vi "FA Forces View.vi"(11 "Model in":refnum<class "Model.lvclass">) -> ()   [LabVIEW 2016, in "M1M3SupportEUI_Views.lvlib"]
uses:
  M1M3SupportEUI_Views.lvlib
  Model/Model.lvclass
  M1M3 Support Events/M1M3 Support Events.lvclass/M1M3 Support Events.ctl
  SALLV_m1m3/DataTypes/command_ApplyOffsetForces.ctl
  SALLV_m1m3/DataTypes/command_ClearOffsetForces.ctl
  SALLV_m1m3/DataTypes/command_ApplyActiveOpticForces.ctl
  SALLV_m1m3/DataTypes/command_ClearActiveOpticForces.ctl
  SALLV_m1m3/DataTypes/command_ApplyAberrationForces.ctl
  SALLV_m1m3/DataTypes/command_ClearAberrationForces.ctl
  M1M3 Support Events/M1M3 Support Events.lvclass
  EUI Events/EUI Events.lvclass
  SALLV_m1m3/SALLV_m1m3.lvlib
panel:
  in  "ClearAberrationForcesButton":bool
  in  "ApplyAberrationForcesButton":bool
  in  "ClearActiveOpticForcesButton":bool
  in  "ApplyActiveOpticForcesButton":bool
  in  "Z441":sgl
  in  "Z440":sgl
  in  "Z443":sgl
  in  "Z442":sgl
  in  "Z401":sgl
  in  "Z431":sgl
  in  "Z430":sgl
  in  "Z439":sgl
  in  "Z438":sgl
  in  "Z437":sgl
  in  "Z436":sgl
  in  "Z435":sgl
  in  "Z434":sgl
  in  "Z433":sgl
  in  "Z432":sgl
  in  "Z421":sgl
  in  "Z420":sgl
  in  "Z429":sgl
  in  "Z428":sgl
  in  "Z427":sgl
  in  "Z426":sgl
  in  "Z425":sgl
  in  "Z424":sgl
  in  "Z423":sgl
  in  "Z422":sgl
  in  "Z411":sgl
  in  "Z410":sgl
  in  "Z419":sgl
  in  "Z418":sgl
  in  "Z417":sgl
  in  "Z416":sgl
  in  "Z415":sgl
  in  "Z414":sgl
  in  "Z413":sgl
  in  "Z412":sgl
  in  "Z409":sgl
  in  "Z408":sgl
  in  "Z407":sgl
  in  "Z406":sgl
  in  "Z405":sgl
  in  "Z404":sgl
  in  "Z403":sgl
  in  "Z402":sgl
  in  "Z341":sgl
  in  "Z340":sgl
  in  "Z343":sgl
  in  "Z342":sgl
  in  "Z301":sgl
  in  "Z331":sgl
  in  "Z330":sgl
  in  "Z339":sgl
  in  "Z338":sgl
  in  "Z337":sgl
  in  "Z336":sgl
  in  "Z335":sgl
  in  "Z334":sgl
  in  "Z333":sgl
  in  "Z332":sgl
  in  "Z321":sgl
  in  "Z320":sgl
  in  "Z329":sgl
  in  "Z328":sgl
  in  "Z327":sgl
  in  "Z326":sgl
  in  "Z325":sgl
  in  "Z324":sgl
  in  "Z323":sgl
  in  "Z322":sgl
  in  "Z311":sgl
  in  "Z310":sgl
  in  "Z319":sgl
  in  "Z318":sgl
  in  "Z317":sgl
  in  "Z316":sgl
  in  "Z315":sgl
  in  "Z314":sgl
  in  "Z313":sgl
  in  "Z312":sgl
  in  "Z309":sgl
  in  "Z308":sgl
  in  "Z307":sgl
  in  "Z306":sgl
  in  "Z305":sgl
  in  "Z304":sgl
  in  "Z303":sgl
  in  "Z302":sgl
  in  "Z241":sgl
  in  "Z240":sgl
  in  "Z243":sgl
  in  "Z242":sgl
  in  "Z201":sgl
  in  "Z231":sgl
  in  "Z230":sgl
  in  "Z239":sgl
  in  "Z238":sgl
  in  "Z237":sgl
  in  "Z236":sgl
  in  "Z235":sgl
  in  "Z234":sgl
  in  "Z233":sgl
  in  "Z232":sgl
  in  "Z221":sgl
  in  "Z220":sgl
  in  "Z229":sgl
  in  "Z228":sgl
  in  "Z227":sgl
  in  "Z226":sgl
  in  "Z225":sgl
  in  "Z224":sgl
  in  "Z223":sgl
  in  "Z222":sgl
  in  "Z211":sgl
  in  "Z210":sgl
  in  "Z219":sgl
  in  "Z218":sgl
  in  "Z217":sgl
  in  "Z216":sgl
  in  "Z215":sgl
  in  "Z214":sgl
  in  "Z213":sgl
  in  "Z212":sgl
  in  "Z209":sgl
  in  "Z208":sgl
  in  "Z207":sgl
  in  "Z206":sgl
  in  "Z205":sgl
  in  "Z204":sgl
  in  "Z203":sgl
  in  "Z202":sgl
  in  "Y430":sgl
  in  "Y438":sgl
  in  "Y437":sgl
  in  "Y434":sgl
  in  "Y433":sgl
  in  "Y432":sgl
  in  "Y421":sgl
  in  "Y420":sgl
  in  "Y429":sgl
  in  "Y427":sgl
  in  "Y424":sgl
  in  "Y423":sgl
  in  "Y422":sgl
  in  "Y411":sgl
  in  "Y410":sgl
  in  "Y418":sgl
  in  "Y417":sgl
  in  "Y416":sgl
  in  "Y415":sgl
  in  "Y414":sgl
  in  "Y409":sgl
  in  "Y408":sgl
  in  "Y230":sgl
  in  "Y238":sgl
  in  "Y237":sgl
  in  "Y234":sgl
  in  "Y233":sgl
  in  "Y232":sgl
  in  "Y221":sgl
  in  "Y220":sgl
  in  "Y229":sgl
  in  "Y227":sgl
  in  "Y224":sgl
  in  "Y223":sgl
  in  "Y222":sgl
  in  "Y211":sgl
  in  "Y210":sgl
  in  "Y218":sgl
  in  "Y217":sgl
  in  "Y216":sgl
  in  "Y215":sgl
  in  "Y214":sgl
  in  "Y209":sgl
  in  "Y208":sgl
  in  "Y330":sgl
  in  "Y338":sgl
  in  "Y337":sgl
  in  "Y334":sgl
  in  "Y333":sgl
  in  "Y332":sgl
  in  "Y321":sgl
  in  "Y320":sgl
  in  "Y329":sgl
  in  "Y327":sgl
  in  "Y326":sgl
  in  "Y324":sgl
  in  "Y323":sgl
  in  "Y322":sgl
  in  "Y311":sgl
  in  "Y310":sgl
  in  "Y318":sgl
  in  "Y317":sgl
  in  "Y316":sgl
  in  "Y315":sgl
  in  "Y314":sgl
  in  "Y313":sgl
  in  "Y309":sgl
  in  "Y308":sgl
  in  "Y305":sgl
  in  "Y304":sgl
  in  "Y303":sgl
  in  "Y302":sgl
  in  "Z141":sgl
  in  "Z140":sgl
  in  "Z143":sgl
  in  "Z142":sgl
  in  "Z101":sgl
  in  "Z131":sgl
  in  "Z130":sgl
  in  "Z139":sgl
  in  "Z138":sgl
  in  "Z137":sgl
  in  "Z136":sgl
  in  "Z135":sgl
  in  "Z134":sgl
  in  "Z133":sgl
  in  "Z132":sgl
  in  "Z121":sgl
  in  "Z120":sgl
  in  "Z129":sgl
  in  "Z128":sgl
  in  "Z127":sgl
  in  "Z126":sgl
  in  "Z125":sgl
  in  "Z124":sgl
  in  "Z123":sgl
  in  "Z122":sgl
  in  "Z111":sgl
  in  "Z110":sgl
  in  "Z119":sgl
  in  "Z118":sgl
  in  "Z117":sgl
  in  "Z116":sgl
  in  "Z115":sgl
  in  "Z114":sgl
  in  "Z113":sgl
  in  "Z112":sgl
  in  "Z109":sgl
  in  "Z108":sgl
  in  "Z107":sgl
  in  "Z106":sgl
  in  "Z105":sgl
  in  "Z104":sgl
  in  "Z103":sgl
  in  "Z102":sgl
  in  "Y130":sgl
  in  "Y138":sgl
  in  "Y137":sgl
  in  "Y134":sgl
  in  "Y133":sgl
  in  "Y132":sgl
  in  "Y121":sgl
  in  "Y120":sgl
  in  "Y129":sgl
  in  "Y127":sgl
  in  "Y126":sgl
  in  "Y124":sgl
  in  "Y123":sgl
  in  "Y122":sgl
  in  "Y111":sgl
  in  "Y110":sgl
  in  "Y118":sgl
  in  "Y117":sgl
  in  "Y116":sgl
  in  "Y115":sgl
  in  "Y114":sgl
  in  "Y113":sgl
  in  "Y109":sgl
  in  "Y108":sgl
  in  "Y105":sgl
  in  "Y104":sgl
  in  "Y103":sgl
  in  "ClearForcesButton":bool
  in  "ApplyOffsetForcesButton":bool
  in  "Y102":sgl
  in  "X435":sgl
  in  "X428":sgl
  in  "X412":sgl
  in  "X335":sgl
  in  "X328":sgl
  in  "X312":sgl
  in  "X235":sgl
  in  "X228":sgl
  in  "X212":sgl
  in  "X135":sgl
  in  "X128":sgl
  in  "X112":sgl
  # "Force Actuator\nApply Forces"
  # "Z"
  # "Y"
  # "0"
  # "1"
  # "2"
  # "3"
  # "4"
  # "5"
  # "6"
  # "7"
  # "8"
  # "9"
  # "0"
  # "1"
  # "2"
  # "3"
  # "4"
  # "5"
  # "6"
  # "7"
  # "8"
  # "9"
  # "100"
  # "100"
  # "110"
  # "110"
  # "X"
  # "120"
  # "120"
  # "112"
  # "212"
  # "130"
  # "130"
  # "128"
  # "228"
  # "140"
  # "140"
  # "135"
  # "235"
  # "200"
  # "200"
  # "210"
  # "312"
  # "210"
  # "412"
  # "220"
  # "220"
  # "328"
  # "428"
  # "230"
  # "230"
  # "335"
  # "435"
  # "240"
  # "240"
  # "300"
  # "300"
  # "310"
  # "310"
  # "320"
  # "320"
  # "330"
  # "330"
  # "340"
  # "340"
  # "400"
  # "400"
  # "410"
  # "410"
  # "420"
  # "420"
  # "430"
  # "430"
  # "440"
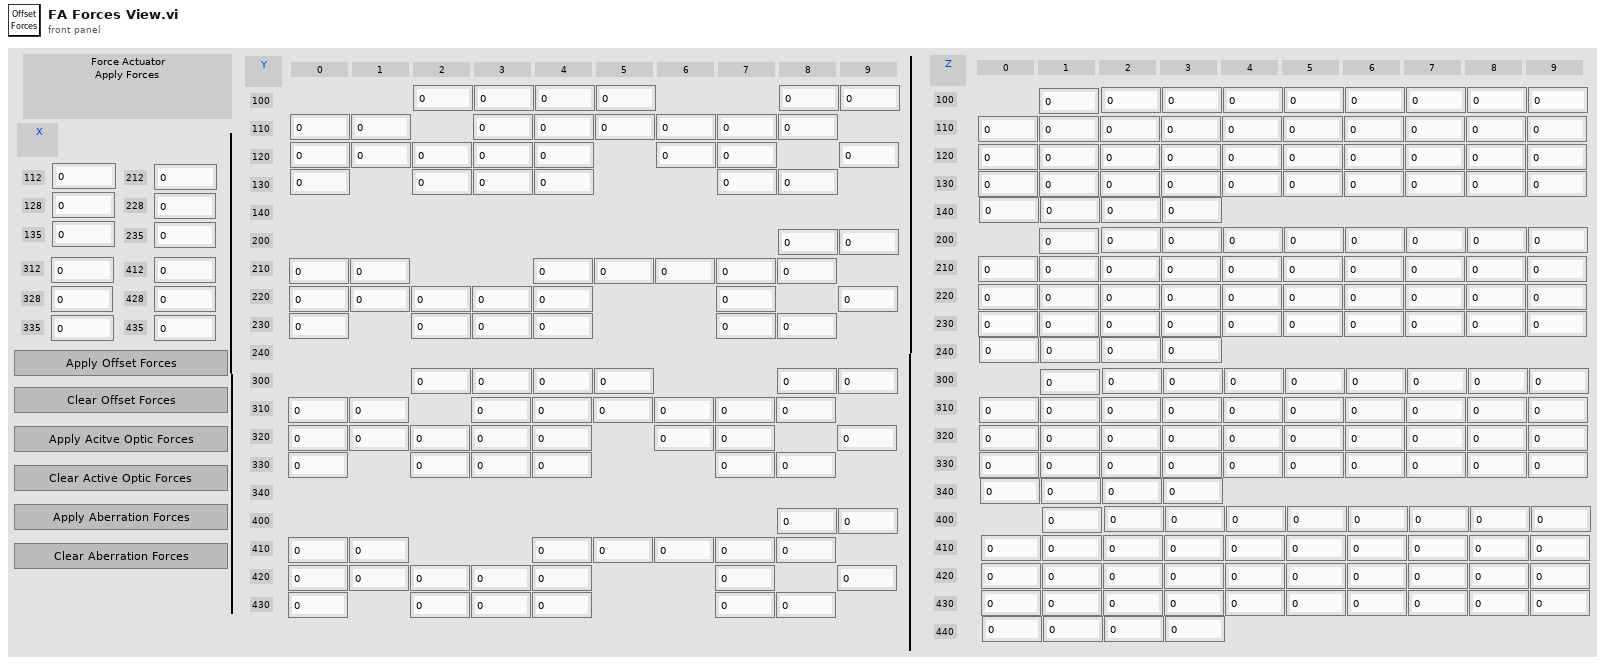
[diagram p1: front panel]
types:
  T1 = typedef "M1M3SupportEUI_TypeDefs.lvlib/M1M3 Support Events.ctl" = cluster{"Inclinometer  Data":refnum<user-event>, "IMS Data":refnum<user-event>, "SAL Connected":refnum<user-event>, "Accelerometer Data":refnum<user-event>, "OuterLoop Data":refnum<user-event>, "ErrorCode Event":refnum<user-event>, "InterlockStatus Event":refnum<user-event>, "InterlockWarning Event":refnum<user-event>, "Gyro Data":refnum<user-event>, "HP Actuator Info Event":refnum<user-event>, " FA Info Event":refnum<user-event>, "HP Monitor Info Event":refnum<user-event>, "FA Data":refnum<user-event>, "HP Actuator data":refnum<user-event>, "HP Monitor data":refnum<user-event>, "Air Supply Status Event":refnum<user-event>, "Air Supply Warning Event":refnum<user-event>, "Power Data":refnum<user-event>, "PID Data":refnum<user-event>, "PID Info Event":refnum<user-event>, "Power Status Event":refnum<user-event>, "Power Supply Status Event":refnum<user-event>, "Power Warning Event":refnum<user-event>, "Summary State Event":refnum<user-event>, "Detailed State Event":refnum<user-event>, "FA Force Warning Event":refnum<user-event>, "FA Warning Event":refnum<user-event>, "FA State Event":refnum<user-event>, "Applied AberrationForces Event":refnum<user-event>, "Applied Acceleration Forcces Event":refnum<user-event>, "Applied Azimuth Forces Event":refnum<user-event>, "Applied Active Optic Forces Event":refnum<user-event>, "Applied Balance Forces Event":refnum<user-event>, "Applied Cylinder Forces Event":refnum<user-event>, "Applied Elevation Forces Event":refnum<user-event>, "Applied Forces Event":refnum<user-event>, "Applied Offset Forces Event":refnum<user-event>, "Applied Static Forces Event":refnum<user-event>, "Applied Thermal Forces Event":refnum<user-event>, "Applied Velocity Forces Event":refnum<user-event>, "Rejected Aberration Force Event":refnum<user-event>, "Rejected Acceleration Forces Event":refnum<user-event>, "Rejected Active Optic Forces Event":refnum<user-event>, "Rejected Azimuth Forces Event":refnum<user-event>, "Rejected Balance Forces Event":refnum<user-event>, "Rejected Cylinder Forces Event":refnum<user-event>, "Rejected Elevation Forces Event":refnum<user-event>, "Rejected Forces Event":refnum<user-event>, "Rejected Offset Forces Event":refnum<user-event>, "Rejected Static Forces Event":refnum<user-event>, "Rejected Thermal Forces Event":refnum<user-event>, "Rejected Velocity Forces Event":refnum<user-event>, "Command Rejection Event":refnum<user-event>, "Setting Verions Event":refnum<user-event>, "Settings Applied Event":refnum<user-event>}
  T2 = enum16{"", "DetailedState_DetailedStates_DisabledState", "DetailedState_DetailedStates_EnabledState", "DetailedState_DetailedStates_FaultState", "DetailedState_DetailedStates_OfflineState", "DetailedState_DetailedStates_StandbyState", "DetailedState_DetailedStates_ParkedState", "DetailedState_DetailedStates_RaisingState", "DetailedState_DetailedStates_ActiveState", "DetailedState_DetailedStates_LoweringState", "DetailedState_DetailedStates_EngineeringState", "DetailedState_DetailedStates_ParkedEngineeringState", "DetailedState_DetailedStates_RaisingEngineeringState", "DetailedState_DetailedStates_ActiveEngineeringState", "DetailedState_DetailedStates_LoweringEngineeringState", "DetailedState_DetailedStates_LoweringFaultState", "DetailedState_DetailedStates_ProfileHardpointCorrectionState"}
  T3 = typedef "SALLV_m1m3.lvlib/command_ApplyOffsetForces.ctl" = cluster{"XForces[12]":sgl[], "YForces[100]":sgl[], "ZForces[156]":sgl[]}
  T4 = typedef "SALLV_m1m3.lvlib/command_ClearOffsetForces.ctl" = cluster{"ClearOffsetForces":bool}
  T5 = typedef "SALLV_m1m3.lvlib/command_ApplyActiveOpticForces.ctl" = cluster{"ZForces[156]":sgl[]}
  T6 = typedef "SALLV_m1m3.lvlib/command_ClearActiveOpticForces.ctl" = cluster{"ClearActiveOpticForces":bool}
  T7 = typedef "SALLV_m1m3.lvlib/command_ApplyAberrationForces.ctl" = cluster{"ZForces[156]":sgl[]}
  T8 = typedef "SALLV_m1m3.lvlib/command_ClearAberrationForces.ctl" = cluster{"ClearAberrationForces":bool}
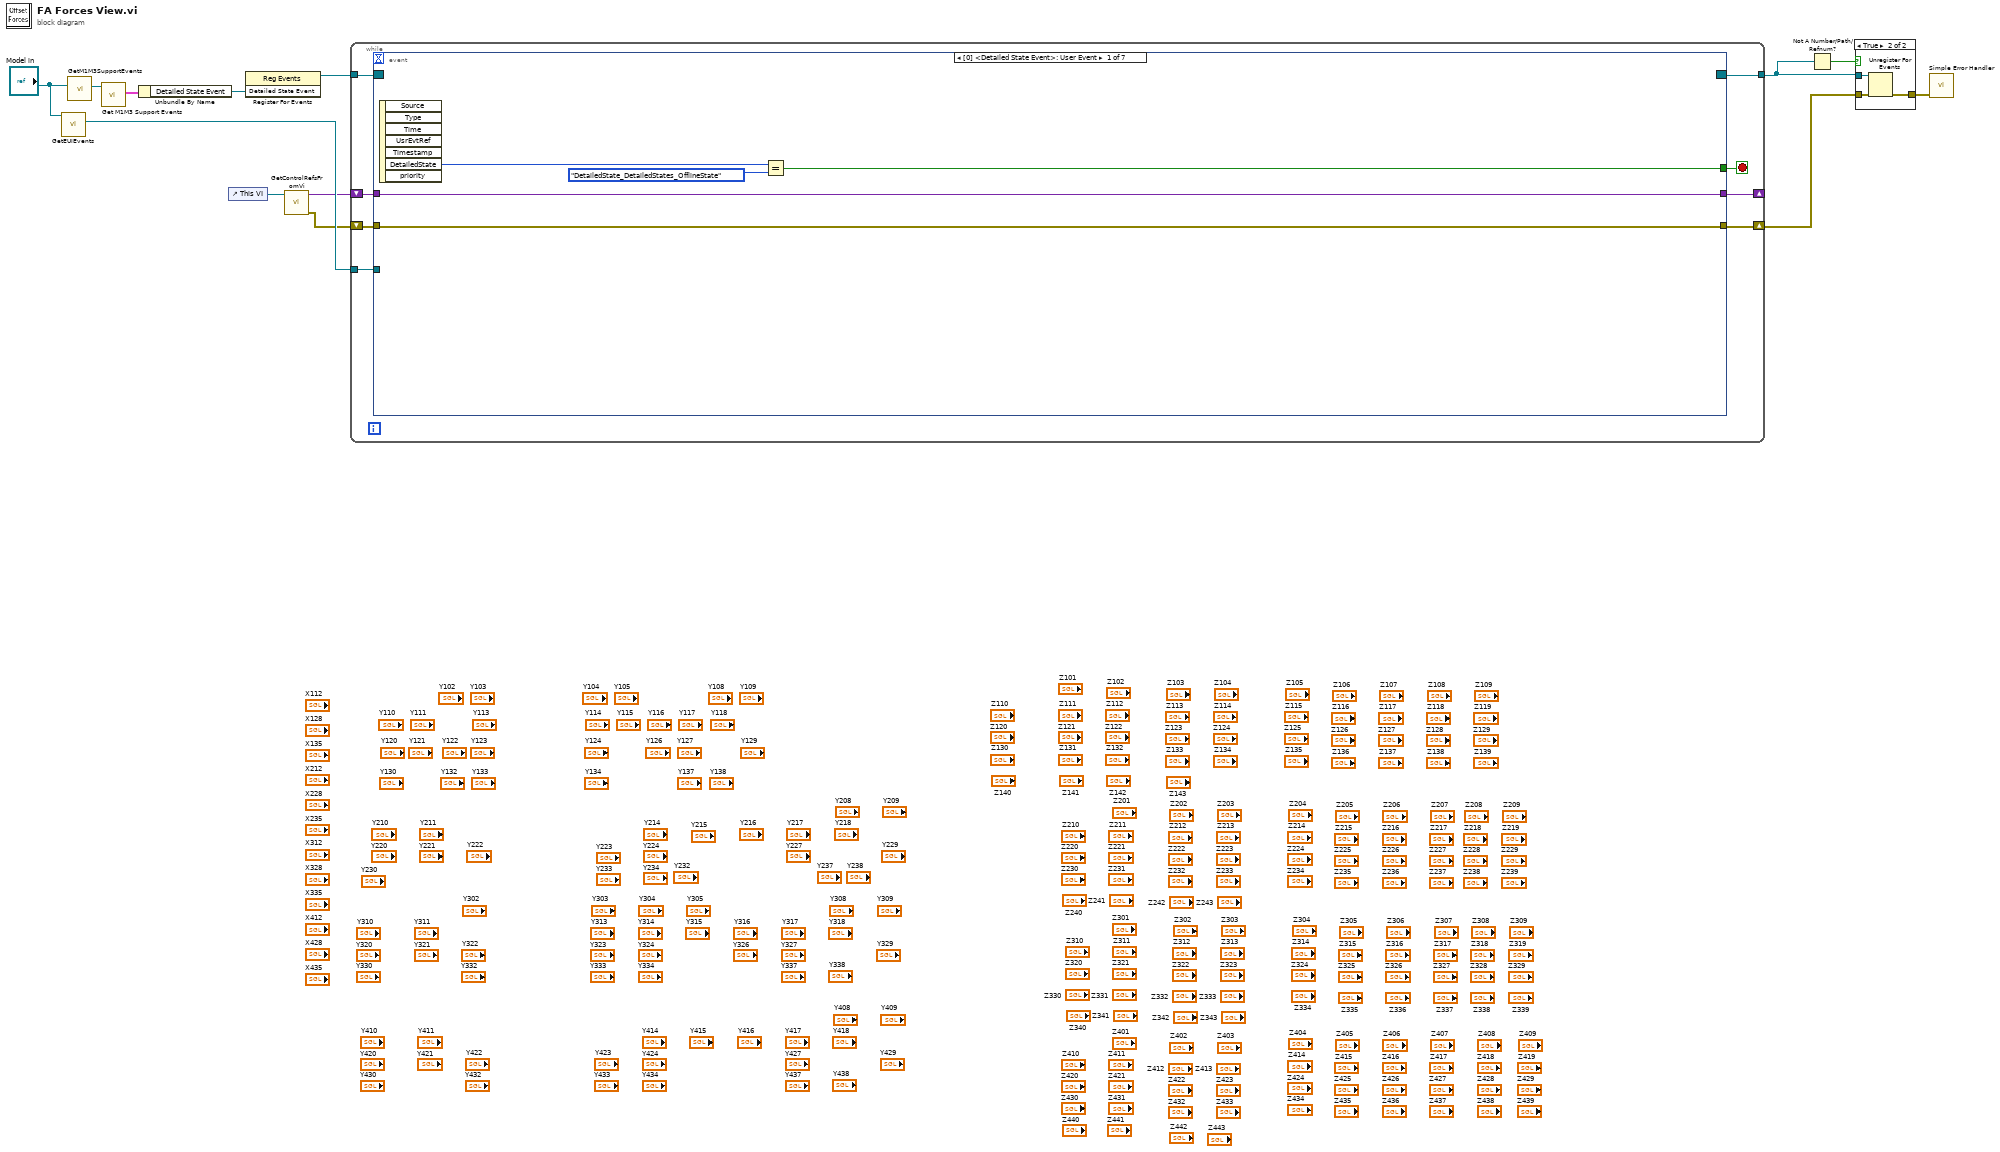
[diagram p0: block diagram]
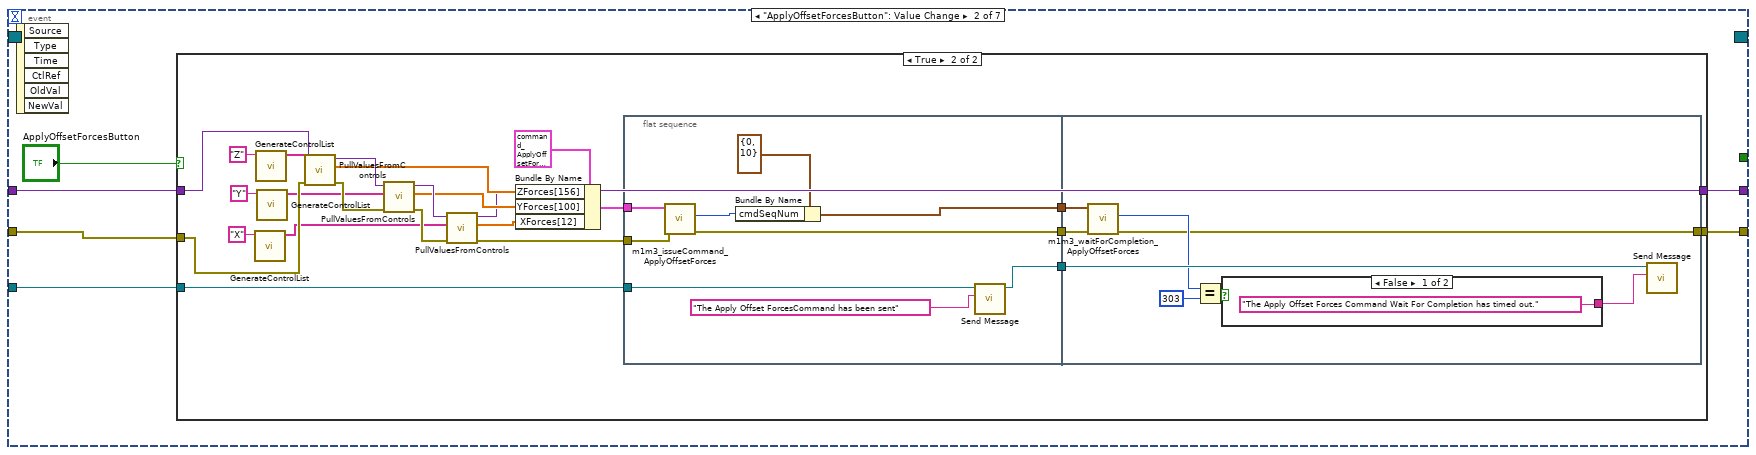
[diagram p2: hidden frame]
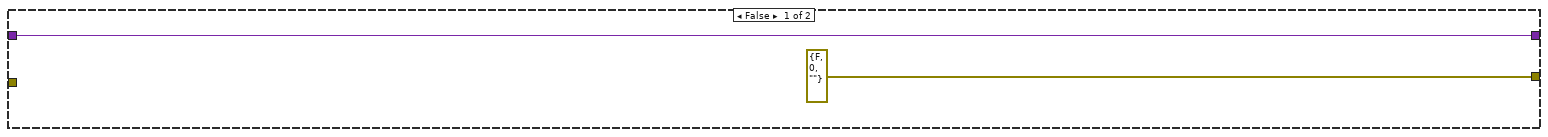
[diagram p3: hidden frame]
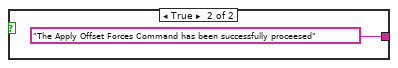
[diagram p4: hidden frame]
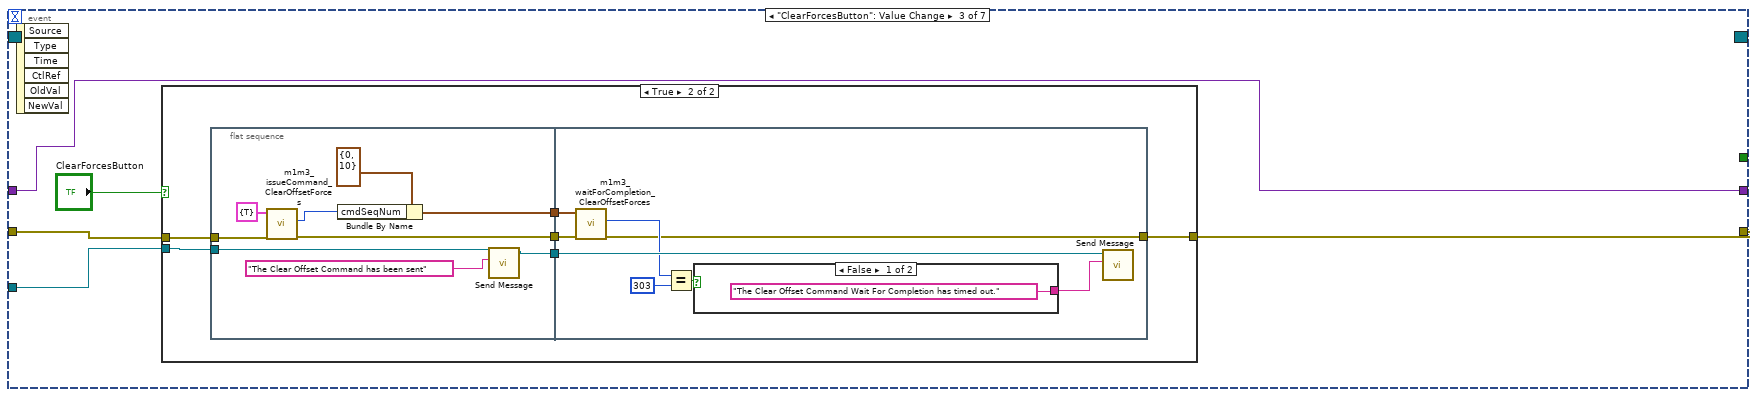
[diagram p5: hidden frame]
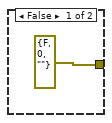
[diagram p6: hidden frame]
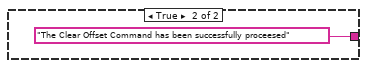
[diagram p7: hidden frame]
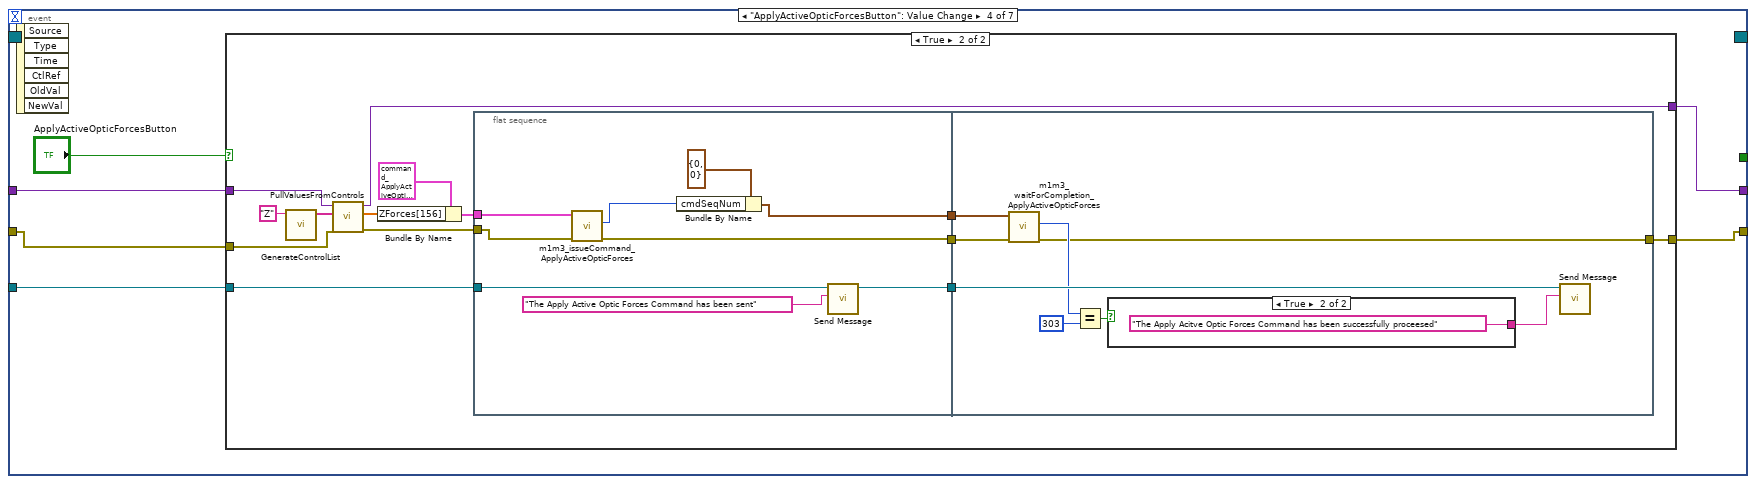
[diagram p8: hidden frame]
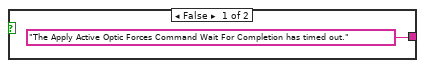
[diagram p10: hidden frame]
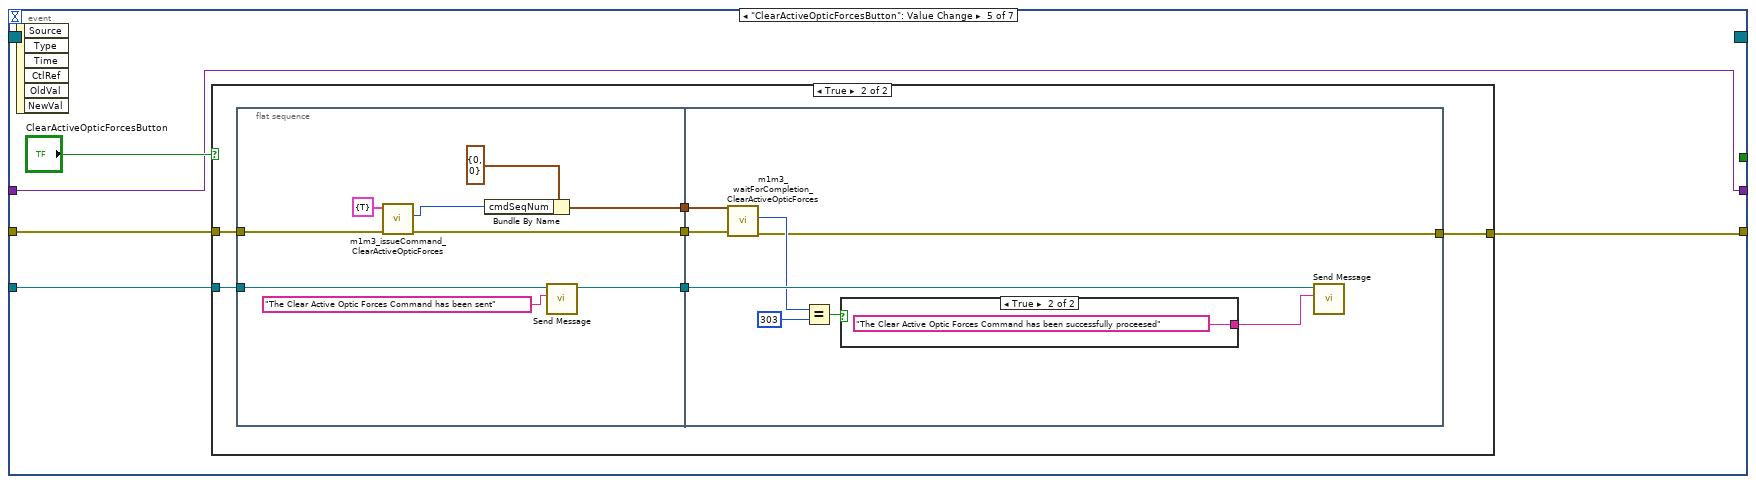
[diagram p11: hidden frame]
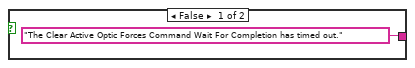
[diagram p13: hidden frame]
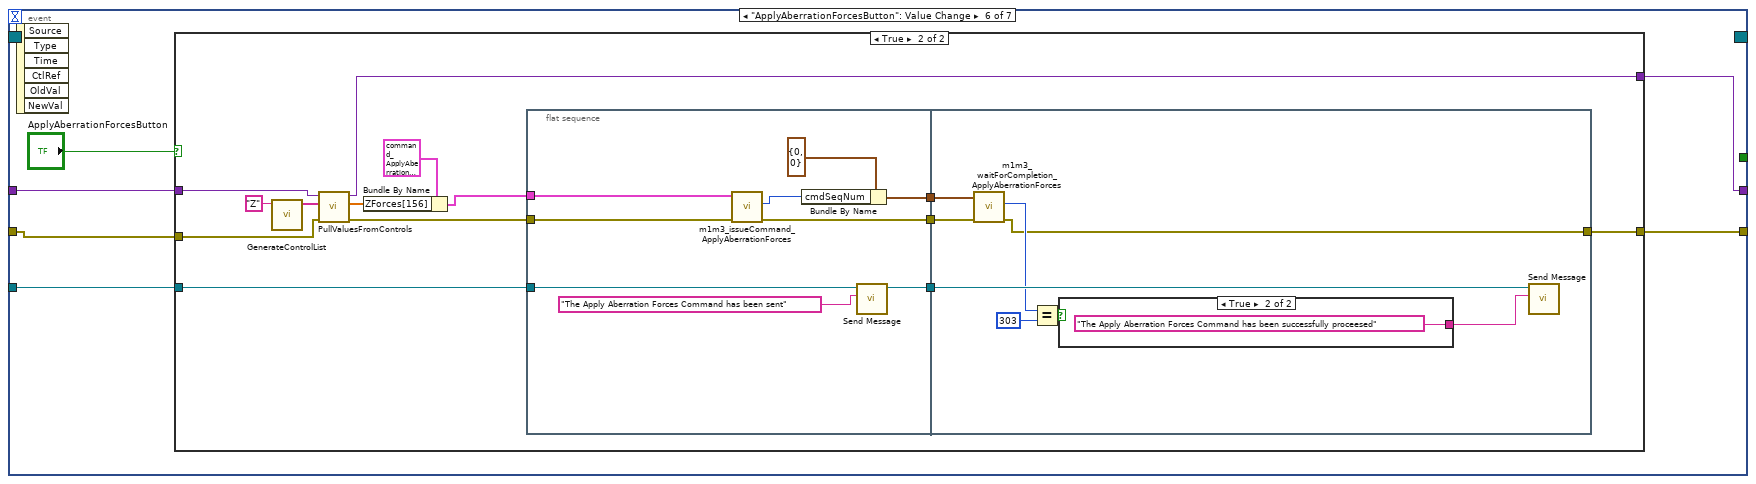
[diagram p14: hidden frame]
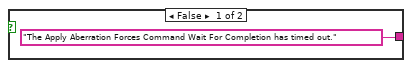
[diagram p16: hidden frame]
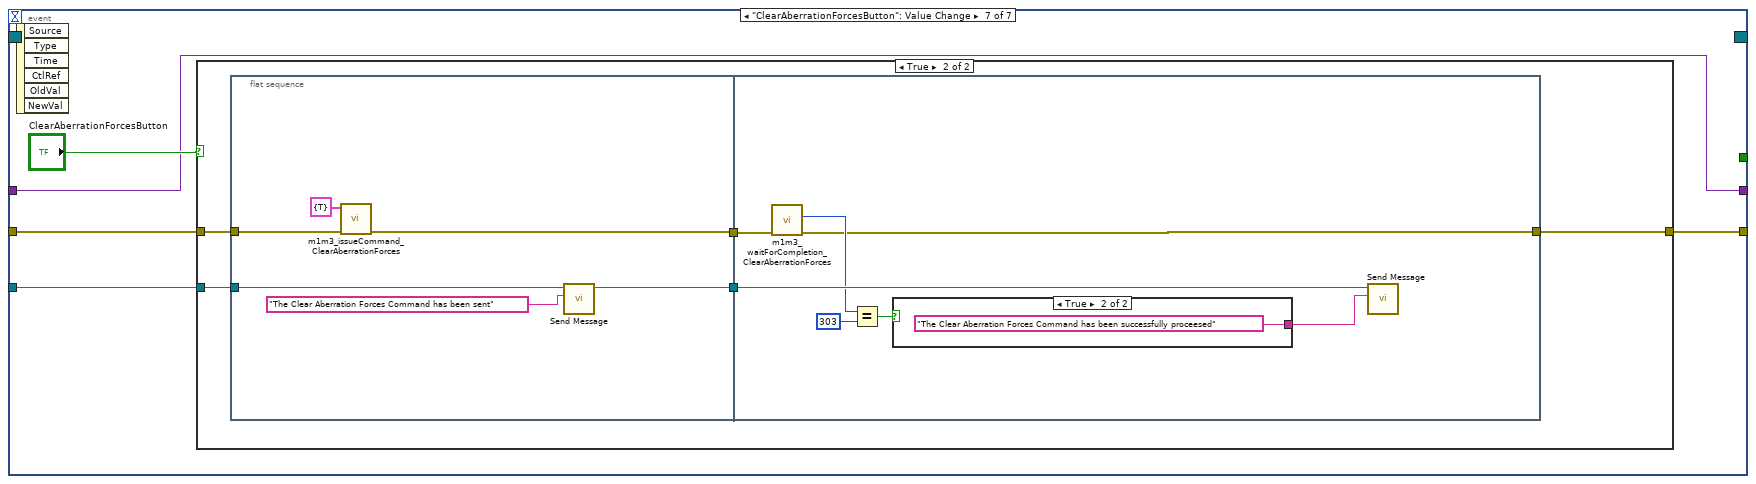
[diagram p17: hidden frame]
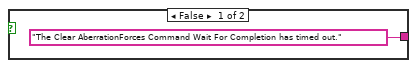
[diagram p19: hidden frame]
diagram:
  n1 = call "GetEUIEvents.vi"("Model in"="Model in") -> ("EUI Events out"=w5:refnum<class "EUI Events.lvclass">)  [unwired: 8 in, 2 out]
  n2 = call "GetM1M3SupportEvents.vi"("Model in"="Model in") -> ("M1M3 Support Events out"=w12:refnum<class "M1M3 Support Events.lvclass">)  [unwired: 8 in, 2 out]
  n3 = call "Get M1M3 Support Events.vi"("M1M3 Support Events in"=w12) -> ("M1M3 Support Events"=w11:T1)  [unwired: 9 in, 1 out]
  n4 = Unbundle By Name(w11) -> ("Detailed State Event"=w13:refnum<user-event>)
  n5 = control-ref of="This VI"() -> (w3:refnum<vi>)
  n6 = register-events(w13) -> (reference out=w10:refnum<event-registration>)  [unwired: 2 in, 1 out]
  n7 = call "GetControlRefsFromVi.vi"("VI Refnum"=w3) -> ("error out"=w1:errorcluster, "Variant"=w2:variant)  [unwired: 9 in]
  n8 = while {
    tunnel: w10 -> [w21]
    tunnel: [w20] -> w7
    tunnel: w5 -> [w18]
    shift-right: [w15] -> _
    shift-left: w2 -> [w17]
    shift-right: [w14] -> w4
    shift-left: w1 -> [w16]
    stop <- w19 stop-if-true
    n9 = event shown="[0] <Detailed State Event>: User Event" {
      selector: w21 -> [_ _ _ _ _ _ _]
      dyn-events: [_ _ _ _ _ _ _] -> w20
      timeout: _ -> [_ _ _ _ _ _ _]
      tunnel: [w24 _ _ _ _ _ _] -> w19
      tunnel: w18 -> [_ w31 w81 w111 w152 w185 w225]
      tunnel: [w22 w30 w80 w109 w150 w182 w222] -> w14
      tunnel: w17 -> [w23 w29 w79 w113 w153 w184 w224]
      tunnel: w16 -> [w22 w28 w78 w112 w151 w183 w223]
      tunnel: [w23 w27 w79 w110 w153 w181 w224] -> w15
      event User Event {
        n10 = event-data() -> ("DetailedState"=w25:T2)  [unwired: 1 in, 6 out]
        n11 = Equal?(x=w25, y=T2."DetailedState_DetailedStates_OfflineState") -> (x = y?=w24:bool)
      }
      event "ApplyOffsetForcesButton": Value Change {
        n12 = event-data() -> ()  [unwired: 1 in, 6 out]
        n13 = case shown="True" "ApplyOffsetForcesButton" {
          tunnel: w31 -> [_ w58]
          tunnel: [errorcluster {"status"=FALSE, "code"=0, "source"=""} ("error constant") w52] -> w30
          tunnel: w29 -> [w33 w51]
          tunnel: w28 -> [_ w50]
          tunnel: [w33 w41] -> w27
          frame False {
          }
          frame True {
            n14 = call "GenerateControlList.vi"("ListType"="X") -> ("ControlList"=w35:string[])  [unwired: 10 in]
            n15 = call "GenerateControlList.vi"("ListType"="Z") -> ("ControlList"=w37:string[])  [unwired: 10 in]
            n16 = call "GenerateControlList.vi"("ListType"="Y") -> ("ControlList"=w36:string[])  [unwired: 10 in]
            n17 = call "PullValuesFromControls.vi"("error in (no error)"=w50, "ControlNameArray"=w37, "Variant In"=w51) -> ("error out"=w48:errorcluster, "ControlValuesArray"=w43:sgl[], "Variant out"=w49:variant)  [unwired: 6 in]
            n18 = call "PullValuesFromControls.vi"("error in (no error)"=w48, "ControlNameArray"=w36, "Variant In"=w49) -> ("error out"=w47:errorcluster, "ControlValuesArray"=w44:sgl[], "Variant out"=w46:variant)  [unwired: 6 in]
            n19 = call "PullValuesFromControls.vi"("error in (no error)"=w47, "ControlNameArray"=w35, "Variant In"=w46) -> ("error out"=w42:errorcluster, "ControlValuesArray"=w45:sgl[], "Variant out"=w41:variant)  [unwired: 6 in]
            n20 = Bundle By Name(cluster=T3 {"XForces[12]"=[0.0, 0.0, 0.0, 0.0, 0.0, 0.0, 0.0, 0.0, 0.0, 0.0, 0.0, 0.0], "YForces[100]"=[0.0, 0.0, 0.0, 0.0, 0.0, 0.0, 0.0, 0.0, 0.0, 0.0, 0.0, 0.0, 0.0, 0.0, 0.0, 0.0, 0.0, 0.0, 0.0, 0.0, 0.0, 0.0, 0.0, 0.0, 0.0, 0.0, 0.0, 0.0, 0.0, 0.0, 0.0, 0.0, 0.0, 0.0, 0.0, 0.0, 0.0, 0.0, 0.0, 0.0, 0.0, 0.0, 0.0, 0.0, 0.0, 0.0, 0.0, 0.0, 0.0, 0.0, 0.0, 0.0, 0.0, 0.0, 0.0, 0.0, 0.0, 0.0, 0.0, 0.0, 0.0, 0.0, 0.0, 0.0, 0.0, 0.0, 0.0, 0.0, 0.0, 0.0, 0.0, 0.0, 0.0, 0.0, 0.0, 0.0, 0.0, 0.0, 0.0, 0.0, 0.0, 0.0, 0.0, 0.0, 0.0, 0.0, 0.0, 0.0, 0.0, 0.0, 0.0, 0.0, 0.0, 0.0, 0.0, 0.0, 0.0, 0.0, 0.0, 0.0], "ZForces[156]"=[0.0, 0.0, 0.0, 0.0, 0.0, 0.0, 0.0, 0.0, 0.0, 0.0, 0.0, 0.0, 0.0, 0.0, 0.0, 0.0, 0.0, 0.0, 0.0, 0.0, 0.0, 0.0, 0.0, 0.0, 0.0, 0.0, 0.0, 0.0, 0.0, 0.0, 0.0, 0.0, 0.0, 0.0, 0.0, 0.0, 0.0, 0.0, 0.0, 0.0, 0.0, 0.0, 0.0, 0.0, 0.0, 0.0, 0.0, 0.0, 0.0, 0.0, 0.0, 0.0, 0.0, 0.0, 0.0, 0.0, 0.0, 0.0, 0.0, 0.0, 0.0, 0.0, 0.0, 0.0, 0.0, 0.0, 0.0, 0.0, 0.0, 0.0, 0.0, 0.0, 0.0, 0.0, 0.0, 0.0, 0.0, 0.0, 0.0, 0.0, 0.0, 0.0, 0.0, 0.0, 0.0, 0.0, 0.0, 0.0, 0.0, 0.0, 0.0, 0.0, 0.0, 0.0, 0.0, 0.0, 0.0, 0.0, 0.0, 0.0, 0.0, 0.0, 0.0, 0.0, 0.0, 0.0, 0.0, 0.0, 0.0, 0.0, 0.0, 0.0, 0.0, 0.0, 0.0, 0.0, 0.0, 0.0, 0.0, 0.0, 0.0, 0.0, 0.0, 0.0, 0.0, 0.0, 0.0, 0.0, 0.0, 0.0, 0.0, 0.0, 0.0, 0.0, 0.0, 0.0, 0.0, 0.0, 0.0, 0.0, 0.0, 0.0, 0.0, 0.0, 0.0, 0.0, 0.0, 0.0, 0.0, 0.0, 0.0, 0.0, 0.0, 0.0, 0.0, 0.0]} ("command_ApplyOffsetForces_Ctl"), "ZForces[156]"=w43, "YForces[100]"=w44, "XForces[12]"=w45) -> (w55:T3)
            n21 = flat-sequence {
              tunnel: w58 -> [w67]
              tunnel: [w65] -> w57
              tunnel: w55 -> [w64]
              tunnel: w42 -> [w63]
              tunnel: [w60] -> w54
              tunnel: [w59] -> w53
              tunnel: w57 -> [w72]
              tunnel: w54 -> [w71]
              tunnel: w53 -> [w70]
              tunnel: [w68] -> w52
              frame #0 {
                n22 = call "m1m3_issueCommand_ApplyOffsetForces.vi"("error in (no error)"=w63, "command_ApplyOffsetForces_Ctl"=w64) -> ("error out"=w60:errorcluster, "function return"=w61:i32)  [unwired: 7 in, 1 out]
                n23 = Bundle By Name(cluster=cluster{"cmdSeqNum":i32, "timeout":u32} {"cmdSeqNum"=0, "timeout"=10} ("waitComplete_Ctl"), "cmdSeqNum"=w61) -> (w59:cluster{"cmdSeqNum":i32, "timeout":u32})
                n24 = call "Send Message.vi"("Message"="The Apply Offset ForcesCommand has been sent", "EUI Events in"=w67) -> ("EUI Events out"=w65:refnum<class "EUI Events.lvclass">)  [unwired: 8 in, 1 out]
              }
              frame #1 {
                n25 = call "m1m3_waitForCompletion_ApplyOffsetForces.vi"("error in (no error)"=w71, "waitComplete_Ctl"=w70) -> ("error out"=w68:errorcluster, "function return"=w69:i32)  [unwired: 7 in, 1 out]
                n26 = Equal?(x=w69, y=303) -> (x = y?=w74:bool)
                n27 = case shown="False" w74 {
                  tunnel: ["The Apply Offset Forces Command Wait For Completion has timed out." ("Message") "The Apply Offset Forces Command has been successfully proceesed" ("Message")] -> w73
                  frame False {
                  }
                  frame True {
                  }
                }
                n28 = call "Send Message.vi"("Message"=w73, "EUI Events in"=w72) -> ()  [unwired: 8 in, 2 out]
              }
            }
          }
        }
      }
      event "ClearForcesButton": Value Change {
        n29 = event-data() -> ()  [unwired: 1 in, 6 out]
        n30 = case shown="True" "ClearForcesButton" {
          tunnel: w81 -> [_ w89]
          tunnel: [errorcluster {"status"=FALSE, "code"=0, "source"=""} ("error constant") w85] -> w80
          tunnel: w78 -> [_ w84]
          frame False {
          }
          frame True {
            n31 = flat-sequence {
              tunnel: w89 -> [w97]
              tunnel: [w93] -> w88
              tunnel: [w92] -> w87
              tunnel: [w91] -> w86
              tunnel: w84 -> [w90]
              tunnel: w88 -> [w106]
              tunnel: w87 -> [w105]
              tunnel: w86 -> [w101]
              tunnel: [w99] -> w85
              frame #0 {
                n32 = call "m1m3_issueCommand_ClearOffsetForces.vi"("error in (no error)"=w90, "command_ClearOffsetForces_Ctl"=T4 {"ClearOffsetForces"=TRUE}) -> ("error out"=w93:errorcluster, "function return"=w94:i32)  [unwired: 7 in, 1 out]
                n33 = Bundle By Name(cluster=cluster{"cmdSeqNum":i32, "timeout":u32} {"cmdSeqNum"=0, "timeout"=10} ("waitComplete_Ctl"), "cmdSeqNum"=w94) -> (w92:cluster{"cmdSeqNum":i32, "timeout":u32})
                n34 = call "Send Message.vi"("Message"="The Clear Offset Command has been sent", "EUI Events in"=w97) -> ("EUI Events out"=w91:refnum<class "EUI Events.lvclass">)  [unwired: 8 in, 1 out]
              }
              frame #1 {
                n35 = call "m1m3_waitForCompletion_ClearOffsetForces.vi"("error in (no error)"=w106, "waitComplete_Ctl"=w105) -> ("error out"=w99:errorcluster, "function return"=w100:i32)  [unwired: 7 in, 1 out]
                n36 = Equal?(x=w100, y=303) -> (x = y?=w103:bool)
                n37 = case shown="False" w103 {
                  tunnel: ["The Clear Offset Command Wait For Completion has timed out." ("Message") "The Clear Offset Command has been successfully proceesed" ("Message")] -> w104
                  frame False {
                  }
                  frame True {
                  }
                }
                n38 = call "Send Message.vi"("Message"=w104, "EUI Events in"=w101) -> ()  [unwired: 8 in, 2 out]
              }
            }
          }
        }
      }
      event "ApplyActiveOpticForcesButton": Value Change {
        n39 = event-data() -> ()  [unwired: 1 in, 6 out]
        n40 = case shown="True" "ApplyActiveOpticForcesButton" {
          tunnel: w113 -> [w116 w128]
          tunnel: w112 -> [w115 w127]
          tunnel: w111 -> [_ w124]
          tunnel: [w116 w120] -> w110
          tunnel: [w115 w117] -> w109
          frame False {
          }
          frame True {
            n41 = call "GenerateControlList.vi"("ListType"="Z") -> ("ControlList"=w129:string[])  [unwired: 10 in]
            n42 = call "PullValuesFromControls.vi"("error in (no error)"=w127, "ControlNameArray"=w129, "Variant In"=w128) -> ("error out"=w121:errorcluster, "ControlValuesArray"=w125:sgl[], "Variant out"=w120:variant)  [unwired: 6 in]
            n43 = Bundle By Name(cluster=T5 {"ZForces[156]"=[0.0, 0.0, 0.0, 0.0, 0.0, 0.0, 0.0, 0.0, 0.0, 0.0, 0.0, 0.0, 0.0, 0.0, 0.0, 0.0, 0.0, 0.0, 0.0, 0.0, 0.0, 0.0, 0.0, 0.0, 0.0, 0.0, 0.0, 0.0, 0.0, 0.0, 0.0, 0.0, 0.0, 0.0, 0.0, 0.0, 0.0, 0.0, 0.0, 0.0, 0.0, 0.0, 0.0, 0.0, 0.0, 0.0, 0.0, 0.0, 0.0, 0.0, 0.0, 0.0, 0.0, 0.0, 0.0, 0.0, 0.0, 0.0, 0.0, 0.0, 0.0, 0.0, 0.0, 0.0, 0.0, 0.0, 0.0, 0.0, 0.0, 0.0, 0.0, 0.0, 0.0, 0.0, 0.0, 0.0, 0.0, 0.0, 0.0, 0.0, 0.0, 0.0, 0.0, 0.0, 0.0, 0.0, 0.0, 0.0, 0.0, 0.0, 0.0, 0.0, 0.0, 0.0, 0.0, 0.0, 0.0, 0.0, 0.0, 0.0, 0.0, 0.0, 0.0, 0.0, 0.0, 0.0, 0.0, 0.0, 0.0, 0.0, 0.0, 0.0, 0.0, 0.0, 0.0, 0.0, 0.0, 0.0, 0.0, 0.0, 0.0, 0.0, 0.0, 0.0, 0.0, 0.0, 0.0, 0.0, 0.0, 0.0, 0.0, 0.0, 0.0, 0.0, 0.0, 0.0, 0.0, 0.0, 0.0, 0.0, 0.0, 0.0, 0.0, 0.0, 0.0, 0.0, 0.0, 0.0, 0.0, 0.0, 0.0, 0.0, 0.0, 0.0, 0.0, 0.0]} ("command_ApplyActiveOpticForces"), "ZForces[156]"=w125) -> (w122:T5)
            n44 = flat-sequence {
              tunnel: w124 -> [w138]
              tunnel: [w137] -> w123
              tunnel: w122 -> [w136]
              tunnel: w121 -> [w135]
              tunnel: [w134] -> w119
              tunnel: [w131] -> w118
              tunnel: w123 -> [w144]
              tunnel: w119 -> [w143]
              tunnel: w118 -> [w142]
              tunnel: [w140] -> w117
              frame #0 {
                n45 = call "m1m3_issueCommand_ApplyActiveOpticForces.vi"("error in (no error)"=w135, "command_ApplyActiveOpticForces_Ctl"=w136) -> ("error out"=w134:errorcluster, "function return"=w132:i32)  [unwired: 7 in, 1 out]
                n46 = Bundle By Name(cluster=cluster{"cmdSeqNum":i32, "timeout":u32} {"cmdSeqNum"=0, "timeout"=0} ("waitComplete_Ctl"), "cmdSeqNum"=w132) -> (w131:cluster{"cmdSeqNum":i32, "timeout":u32})
                n47 = call "Send Message.vi"("Message"="The Apply Active Optic Forces Command has been sent", "EUI Events in"=w138) -> ("EUI Events out"=w137:refnum<class "EUI Events.lvclass">)  [unwired: 8 in, 1 out]
              }
              frame #1 {
                n48 = call "m1m3_waitForCompletion_ApplyActiveOpticForces.vi"("error in (no error)"=w143, "waitComplete_Ctl"=w142) -> ("error out"=w140:errorcluster, "function return"=w141:i32)  [unwired: 7 in, 1 out]
                n49 = Equal?(x=w141, y=303) -> (x = y?=w146:bool)
                n50 = case shown="True" w146 {
                  tunnel: ["The Apply Active Optic Forces Command Wait For Completion has timed out." ("Message") "The Apply Acitve Optic Forces Command has been successfully proceesed" ("Message")] -> w147
                  frame False {
                  }
                  frame True {
                  }
                }
                n51 = call "Send Message.vi"("Message"=w147, "EUI Events in"=w144) -> ()  [unwired: 8 in, 2 out]
              }
            }
          }
        }
      }
      event "ClearActiveOpticForcesButton": Value Change {
        n52 = event-data() -> ()  [unwired: 1 in, 6 out]
        n53 = case shown="True" "ClearActiveOpticForcesButton" {
          tunnel: w152 -> [_ w161]
          tunnel: w151 -> [w155 w160]
          tunnel: [w155 w157] -> w150
          frame False {
          }
          frame True {
            n54 = flat-sequence {
              tunnel: w161 -> [w169]
              tunnel: w160 -> [w167]
              tunnel: [w166] -> w159
              tunnel: [w165] -> w158
              tunnel: [w162] -> w156
              tunnel: w159 -> [w174]
              tunnel: w158 -> [w175]
              tunnel: [w172] -> w157
              tunnel: w156 -> [w171]
              frame #0 {
                n55 = call "m1m3_issueCommand_ClearActiveOpticForces.vi"("error in (no error)"=w167, "command_ClearActiveOpticForces_Ctl"=T6 {"ClearActiveOpticForces"=TRUE}) -> ("error out"=w166:errorcluster, "function return"=w163:i32)  [unwired: 7 in, 1 out]
                n56 = Bundle By Name(cluster=cluster{"cmdSeqNum":i32, "timeout":u32} {"cmdSeqNum"=0, "timeout"=0} ("waitComplete_Ctl"), "cmdSeqNum"=w163) -> (w162:cluster{"cmdSeqNum":i32, "timeout":u32})
                n57 = call "Send Message.vi"("Message"="The Clear Active Optic Forces Command has been sent", "EUI Events in"=w169) -> ("EUI Events out"=w165:refnum<class "EUI Events.lvclass">)  [unwired: 8 in, 1 out]
              }
              frame #1 {
                n58 = call "m1m3_waitForCompletion_ClearActiveOpticForces.vi"("error in (no error)"=w174, "waitComplete_Ctl"=w171) -> ("error out"=w172:errorcluster, "function return"=w173:i32)  [unwired: 7 in, 1 out]
                n59 = Equal?(x=w173, y=303) -> (x = y?=w177:bool)
                n60 = case shown="True" w177 {
                  tunnel: ["The Clear Active Optic Forces Command Wait For Completion has timed out." ("Message") "The Clear Active Optic Forces Command has been successfully proceesed" ("Message")] -> w178
                  frame False {
                  }
                  frame True {
                  }
                }
                n61 = call "Send Message.vi"("Message"=w178, "EUI Events in"=w175) -> ()  [unwired: 8 in, 2 out]
              }
            }
          }
        }
      }
      event "ApplyAberrationForcesButton": Value Change {
        n62 = event-data() -> ()  [unwired: 1 in, 6 out]
        n63 = case shown="True" "ApplyAberrationForcesButton" {
          tunnel: w185 -> [_ w202]
          tunnel: w184 -> [w187 w197]
          tunnel: w183 -> [w188 w196]
          tunnel: [w188 w193] -> w182
          tunnel: [w187 w189] -> w181
          frame False {
          }
          frame True {
            n64 = call "GenerateControlList.vi"("ListType"="Z") -> ("ControlList"=w199:string[])  [unwired: 10 in]
            n65 = call "PullValuesFromControls.vi"("error in (no error)"=w196, "ControlNameArray"=w199, "Variant In"=w197) -> ("error out"=w195:errorcluster, "ControlValuesArray"=w198:sgl[], "Variant out"=w189:variant)  [unwired: 6 in]
            n66 = Bundle By Name(cluster=T7 {"ZForces[156]"=[0.0, 0.0, 0.0, 0.0, 0.0, 0.0, 0.0, 0.0, 0.0, 0.0, 0.0, 0.0, 0.0, 0.0, 0.0, 0.0, 0.0, 0.0, 0.0, 0.0, 0.0, 0.0, 0.0, 0.0, 0.0, 0.0, 0.0, 0.0, 0.0, 0.0, 0.0, 0.0, 0.0, 0.0, 0.0, 0.0, 0.0, 0.0, 0.0, 0.0, 0.0, 0.0, 0.0, 0.0, 0.0, 0.0, 0.0, 0.0, 0.0, 0.0, 0.0, 0.0, 0.0, 0.0, 0.0, 0.0, 0.0, 0.0, 0.0, 0.0, 0.0, 0.0, 0.0, 0.0, 0.0, 0.0, 0.0, 0.0, 0.0, 0.0, 0.0, 0.0, 0.0, 0.0, 0.0, 0.0, 0.0, 0.0, 0.0, 0.0, 0.0, 0.0, 0.0, 0.0, 0.0, 0.0, 0.0, 0.0, 0.0, 0.0, 0.0, 0.0, 0.0, 0.0, 0.0, 0.0, 0.0, 0.0, 0.0, 0.0, 0.0, 0.0, 0.0, 0.0, 0.0, 0.0, 0.0, 0.0, 0.0, 0.0, 0.0, 0.0, 0.0, 0.0, 0.0, 0.0, 0.0, 0.0, 0.0, 0.0, 0.0, 0.0, 0.0, 0.0, 0.0, 0.0, 0.0, 0.0, 0.0, 0.0, 0.0, 0.0, 0.0, 0.0, 0.0, 0.0, 0.0, 0.0, 0.0, 0.0, 0.0, 0.0, 0.0, 0.0, 0.0, 0.0, 0.0, 0.0, 0.0, 0.0, 0.0, 0.0, 0.0, 0.0, 0.0, 0.0]} ("command_ApplyAberrationForces"), "ZForces[156]"=w198) -> (w191:T7)
            n67 = flat-sequence {
              tunnel: w202 -> [w210]
              tunnel: [w209] -> w201
              tunnel: w195 -> [w208]
              tunnel: [w207] -> w194
              tunnel: w191 -> [w206]
              tunnel: [w203] -> w190
              tunnel: w201 -> [w216]
              tunnel: w194 -> [w215]
              tunnel: [w213] -> w193
              tunnel: w190 -> [w212]
              frame #0 {
                n68 = call "m1m3_issueCommand_ApplyAberrationForces.vi"("error in (no error)"=w208, "command_ApplyAberrationForces_Ctl"=w206) -> ("error out"=w207:errorcluster, "function return"=w204:i32)  [unwired: 7 in, 1 out]
                n69 = Bundle By Name(cluster=cluster{"cmdSeqNum":i32, "timeout":u32} {"cmdSeqNum"=0, "timeout"=0} ("waitComplete_Ctl"), "cmdSeqNum"=w204) -> (w203:cluster{"cmdSeqNum":i32, "timeout":u32})
                n70 = call "Send Message.vi"("Message"="The Apply Aberration Forces Command has been sent", "EUI Events in"=w210) -> ("EUI Events out"=w209:refnum<class "EUI Events.lvclass">)  [unwired: 8 in, 1 out]
              }
              frame #1 {
                n71 = call "m1m3_waitForCompletion_ApplyAberrationForces.vi"("error in (no error)"=w215, "waitComplete_Ctl"=w212) -> ("error out"=w213:errorcluster, "function return"=w214:i32)  [unwired: 7 in, 1 out]
                n72 = Equal?(x=w214, y=303) -> (x = y?=w218:bool)
                n73 = case shown="True" w218 {
                  tunnel: ["The Apply Aberration Forces Command Wait For Completion has timed out." ("Message") "The Apply Aberration Forces Command has been successfully proceesed" ("Message")] -> w219
                  frame False {
                  }
                  frame True {
                  }
                }
                n74 = call "Send Message.vi"("Message"=w219, "EUI Events in"=w216) -> ()  [unwired: 8 in, 2 out]
              }
            }
          }
        }
      }
      event "ClearAberrationForcesButton": Value Change {
        n75 = event-data() -> ()  [unwired: 1 in, 6 out]
        n76 = case shown="True" "ClearAberrationForcesButton" {
          tunnel: w225 -> [_ w232]
          tunnel: w223 -> [w227 w231]
          tunnel: [w227 w228] -> w222
          frame False {
          }
          frame True {
            n77 = flat-sequence {
              tunnel: w232 -> [w237]
              tunnel: w231 -> [w236]
              tunnel: [w234] -> w230
              tunnel: [w233] -> w229
              tunnel: w230 -> [w245]
              tunnel: w229 -> [w241]
              tunnel: [w239] -> w228
              frame #0 {
                n78 = call "m1m3_issueCommand_ClearAberrationForces.vi"("error in (no error)"=w236, "command_ClearAberrationForces_Ctl"=T8 {"ClearAberrationForces"=TRUE}) -> ("error out"=w234:errorcluster)  [unwired: 7 in, 2 out]
                n79 = call "Send Message.vi"("Message"="The Clear Aberration Forces Command has been sent", "EUI Events in"=w237) -> ("EUI Events out"=w233:refnum<class "EUI Events.lvclass">)  [unwired: 8 in, 1 out]
              }
              frame #1 {
                n80 = call "m1m3_waitForCompletion_ClearAberrationForces.vi"("error in (no error)"=w245) -> ("error out"=w239:errorcluster, "function return"=w240:i32)  [unwired: 8 in, 1 out]
                n81 = Equal?(x=w240, y=303) -> (x = y?=w243:bool)
                n82 = case shown="True" w243 {
                  tunnel: ["The Clear AberrationForces Command Wait For Completion has timed out." ("Message") "The Clear Aberration Forces Command has been successfully proceesed" ("Message")] -> w244
                  frame False {
                  }
                  frame True {
                  }
                }
                n83 = call "Send Message.vi"("Message"=w244, "EUI Events in"=w241) -> ()  [unwired: 8 in, 2 out]
              }
            }
          }
        }
      }
    }
  }
  n84 = Not A Number/Path/Refnum?(number/path/refnum=w7) -> (NaN/Path/Refnum?=w8:bool)
  n85 = case shown="True" w8 {
    tunnel: w7 -> [_ w251]
    tunnel: w4 -> [w248 w250]
    tunnel: [w248 w249] -> w9
    frame False {
    }
    frame True {
      n86 = Unregister For Events(event registration refnum=w251, error in=w250) -> (error out=w249:errorcluster)
    }
  }
  n87 = call <vilib>:"Simple Error Handler.vi"("error in (no error)"=w9) -> ()  [unwired: 4 in, 5 out]
